vi "HP-request.vi"(8 "error in (no error)":errorcluster, 10 "write buffer":T1 format="%x", 11 "HP-S-Serial in":refnum<class "HP-S-Serial.lvclass">) -> (0 "error out":errorcluster, 2 "read buffer":T1 format="%x", 3 "HP-S-Serial out":refnum<class "HP-S-Serial.lvclass">)   [LabVIEW 2020, in "HP-S-Serial.lvclass"]
uses:
  HP-S-Serial.lvclass
  HP-S-data.ctl
  ee36e0e2-efc5-4dac-bd31-cab0864b516f.vi
panel:
  in  "milliseconds to wait":u32=1500
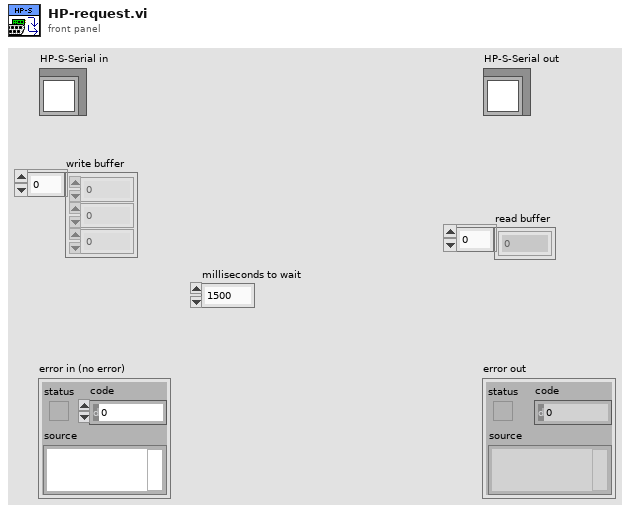
[diagram p1: front panel]
types:
  T1 = typedef "HP-S-Serial.lvclass/HP-S-data.ctl" = u8[]
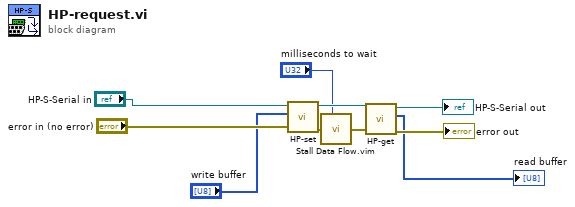
[diagram p0: block diagram]
diagram:
  n1 = call-dynamic "HP-set.vi"("error in (no error)"="error in (no error)", "write buffer"="write buffer", "HP-S-Serial in"="HP-S-Serial in") -> ("error out"=w9:errorcluster, "HP-S-Serial out"=w10:refnum<class "HP-S-Serial.lvclass">)  [unwired: 7 in]
  n2 = call "Stall Data Flow.vim"("value in"=w9, "milliseconds to wait"="milliseconds to wait") -> ("value out"=w2:errorcluster)  [unwired: 1 out]
  n3 = call-dynamic "HP-get.vi"("error in (no error)"=w2, "HP-S-Serial in"=w10) -> ("error out"=→"error out":errorcluster, "read buffer"=→"read buffer":T1, "HP-S-Serial out"=→"HP-S-Serial out":refnum<class "HP-S-Serial.lvclass">)  [unwired: 7 in]
